vi "Stop.vi"(8 "error in (no error)":errorcluster, 10 "Message in":refnum<class "StopMessage.lvclass">, 11 "waveform_FPGA in":refnum<class "waveform_FPGA.lvclass">) -> (0 "error out":errorcluster, 3 "waveform_FPGA out":refnum<class "waveform_FPGA.lvclass">)   [LabVIEW 2012, in "waveform_FPGA.lvclass"]
doc: "This member function is called when the statemachine in the run.vi receives an 'stop' command. It relays the message to all observers of the component.\n\nOverride this member function in your derived class if you need additional stop functionality (but don't forget to call the parent method)."
uses:
  waveform_FPGA.lvclass
  <vilib>/Distrio/Murmex/Murmex/Murmex.lvclass
  <vilib>/Distrio/Murmex/StopMessage/StopMessage.lvclass
panel:
  # "This method is called when the STOP\ntrigger is sent. \n\nOverride this method when your component needs to\nrespond to this trigger. \n\nCall parent for proper implementation"
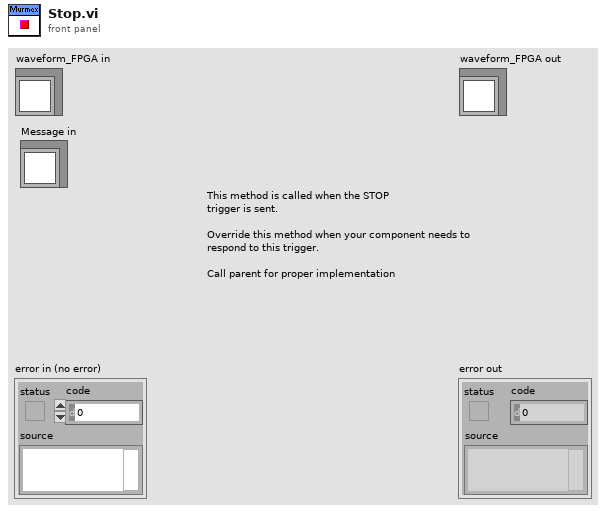
[diagram p1: front panel]
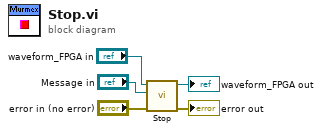
[diagram p0: block diagram]
diagram:
  n1 = call-parent "Stop.vi"("error in (no error)"="error in (no error)", "Message in"="Message in", "Murmex in"="waveform_FPGA in") -> ("error out"=→"error out":errorcluster, "Murmex out"=→"waveform_FPGA out":refnum<class "waveform_FPGA.lvclass">)  [unwired: 7 in]
